vi "Send Message.vi"(8 "error in (no error)":errorcluster, 10 "message":string, 11 "TCS in":refnum<class "TCS.lvclass">) -> (0 "error out":errorcluster, 3 "TCS out":refnum<class "TCS.lvclass">)   [LabVIEW 2018, in "TCS.lvclass"]
uses:
  TCS.lvclass
  TCS.lvclass/TCS.ctl
  RxTx/RxTx.lvclass
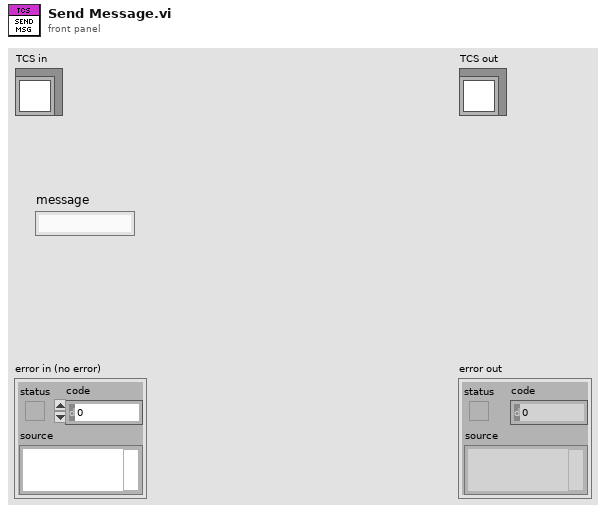
[diagram p1: front panel]
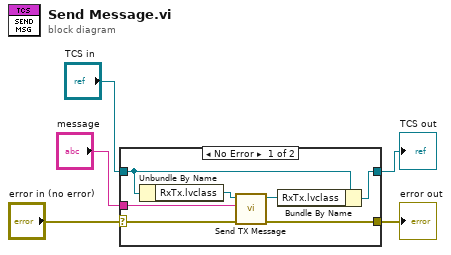
[diagram p0: block diagram]
diagram:
  n1 = case shown="No Error" "error in (no error)" {
    selector: "error in (no error)" -> [w10 w14]
    tunnel: [w7 w14] -> w4
    tunnel: [w11 w13] -> w2
    tunnel: "TCS in" -> [w12 w13]
    tunnel: "message" -> [w6 _]
    frame No Error {
      n2 = Unbundle By Name(w12) -> ("RxTx.lvclass"=w9:refnum<class "RxTx.lvclass">)
      n3 = call "Send TX Message.vi"("error in (no error)"=w10, "element"=w6, "RxTx in"=w9) -> ("error out"=w7:errorcluster, "RxTx out"=w8:refnum<class "RxTx.lvclass">)  [unwired: 7 in]
      n4 = Bundle By Name(cluster=w12, "RxTx.lvclass"=w8) -> (w11:refnum<class "TCS.lvclass">)
    }
    frame Error {
    }
  }
  "error out" <- w4
  "TCS out" <- w2
